vi "Get Common Dependencies.vi"(0 "All dependencies":path[][](array[path]), 11 "error in (no error)":errorcluster) -> (4 "Measurement dependencies":path[][](array[path]), 6 "Measurement index":i32, 8 "Common dependencies":path[](array[path]), 15 "error out":errorcluster)   [LabVIEW 2021, in "Multiple Migrator.lvlib"]
uses:
  Multiple Migrator.lvlib
  29c143f9-24d1-41ec-a67d-85f525be0bbf.vi
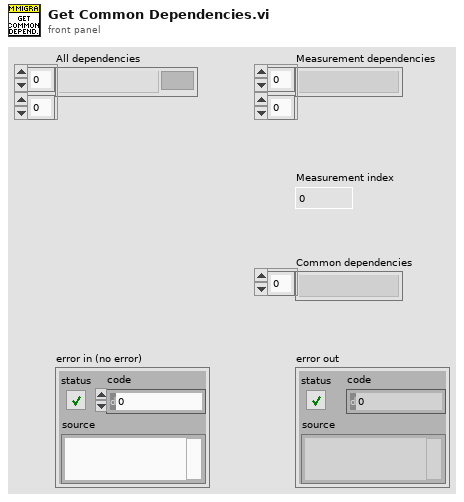
[diagram p1: front panel]
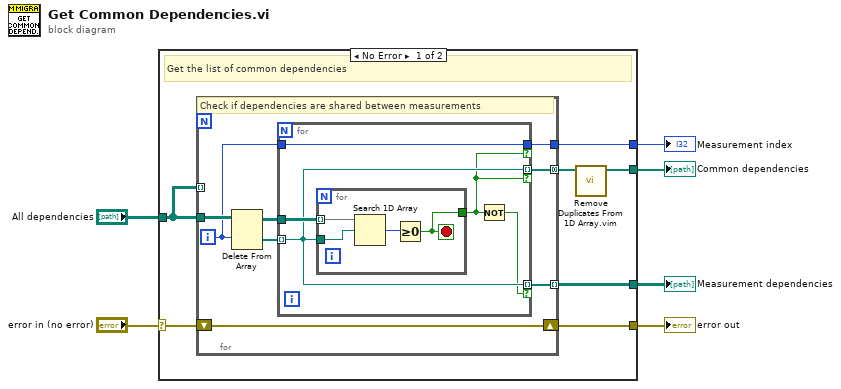
[diagram p0: block diagram]
diagram:
  n1 = case shown="No Error" "error in (no error)" {
    selector: "error in (no error)" -> [w11 w31]
    tunnel: [w13 _] -> w6
    tunnel: [w12 w31] -> w5
    tunnel: "All dependencies" -> [w8 _]
    tunnel: [w9 _] -> w2
    tunnel: [w7 _] -> w1
    frame No Error {
      # "Get the list of common dependencies"
      n2 = for {
        tunnel: [w19] -> w10 mode=concatenating
        tunnel: w8 -> [w18]
        tunnel: [w17] -> w13 mode=indexing
        tunnel: w8 -> [_] mode=indexing
        shift-right: [w16] -> w12
        shift-left: w11 -> [w16]
        tunnel: [w14] -> w7
        i -> [w15]
        # "Check if dependencies are shared between measurements"
        n3 = Delete From Array(array=w18, index (row)=w15) -> (deleted portion=w21:path[], array with subset deleted=w20:path[][])  [unwired: 2 in]
        n4 = for {
          tunnel: w20 -> [w26]
          tunnel: w21 -> [w25] mode=indexing
          tunnel: [w25] -> w19 mode=indexing if=w22
          tunnel: [w25] -> w17 mode=indexing if=w24
          tunnel: [w23] -> w14 if=w22
          tunnel: w15 -> [w23]
          n5 = for {
            tunnel: w25 -> [w28]
            tunnel: w26 -> [w30] mode=indexing
            tunnel: [w27] -> w22
            stop <- w27 stop-if-true
            n6 = Search 1D Array(1D array=w30, element=w28) -> (index of element=w29:i32)  [unwired: 1 in]
            n7 = Greater Or Equal To 0?(x=w29) -> (x >= 0?=w27:bool)
          }
          n8 = Not(x=w22) -> (.not. x?=w24:bool)
        }
      }
      n9 = call "Remove Duplicates From 1D Array.vim"("array"=w10) -> ("array with duplicates removed"=w9:path[])  [unwired: 10 in]
    }
    frame Error {
      # "Pass"
    }
  }
  "Measurement dependencies" <- w6
  "error out" <- w5
  "Common dependencies" <- w2
  "Measurement index" <- w1
